vi "LvMPDC_CMD_Close.vi"(8 "error in (no error)":errorcluster, 11 "Connect ID":refnum<k5>) -> (0 "error out":errorcluster)   [LabVIEW 2012]
panel:
  # "LvMPDC:: Close - DisConnect MPDServer"
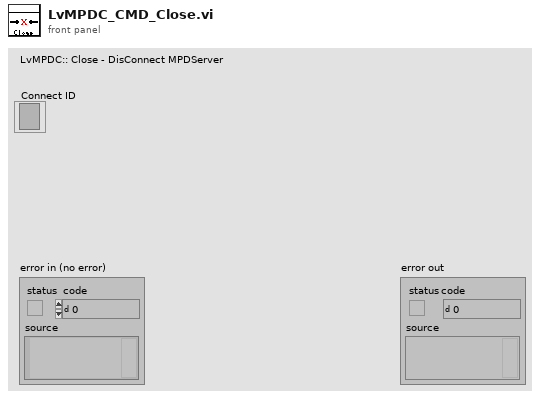
[diagram p1: front panel]
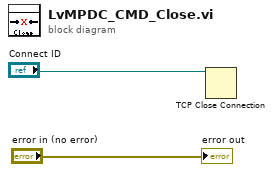
[diagram p0: block diagram]
diagram:
  n1 = TCP Close Connection(connection ID="Connect ID") -> ()  [unwired: 2 in, 2 out]
  "error out" <- "error in (no error)"
